vi "Initialise.vi"(8 "error in (no error)":errorcluster, 10 "Message in":refnum<class "InitialiseMessage.lvclass">, 11 "ImageStack in":refnum<class "ImageStack.lvclass">) -> (0 "error out":errorcluster, 3 "ImageStack out":refnum<class "ImageStack.lvclass">)   [LabVIEW 2012, in "ImageStack.lvclass"]
doc: "This method is called when an initialise message is received. It mainly initialises the RabbitMQ connectivity. \n\nOverride this method when your component needs special initialisation (e.g. of software or hardware resources). In that case, don't forget to call the parent for proper implementation. If your component owns subcomponents, they count as resources, so you have to initialise them by calling their own initialise functions"
uses:
  ImageStack.lvclass
  <vilib>/Distrio/Murmex/InitialiseMessage/InitialiseMessage.lvclass
  <vilib>/Distrio/Murmex/Murmex/Murmex.lvclass
  <vilib>/Distrio/Murmex/Murmex/update_cluster.ctl
  <vilib>/Distrio/Murmex/GenericMessage/GenericMessage.lvclass
  <vilib>/Distrio/Murmex/Message/Add or replace parameter.vi
panel:
  # "This method is called when the INTIALISE\ntrigger is sent. \n\nOverride this method when your component needs to\nrespond to this trigger. \n\nCall parent for proper implementation"
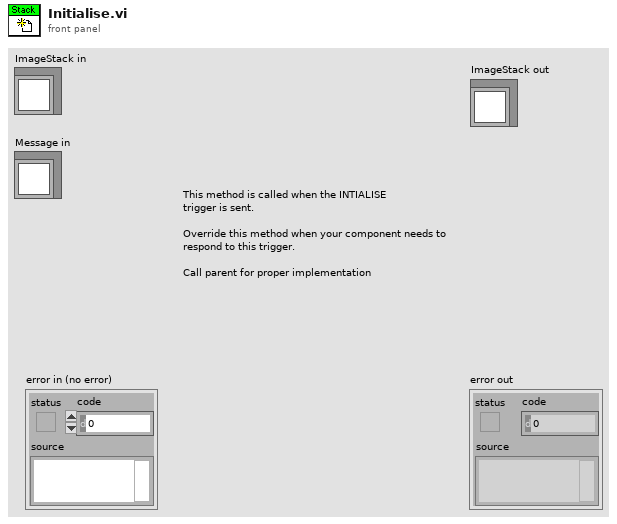
[diagram p1: front panel]
types:
  T1 = typedef "Murmex.lvlib/Murmex.lvclass/update_cluster.ctl" = cluster{"target ID":string, "key chains":string[], "values":variant[]}
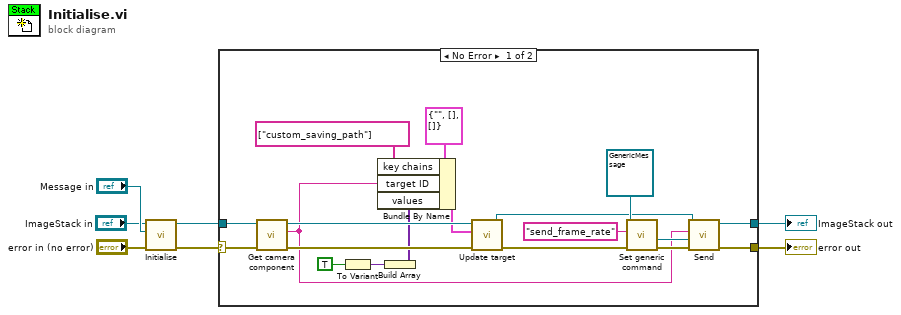
[diagram p0: block diagram]
diagram:
  n1 = call-parent "Initialise.vi"("error in (no error)"="error in (no error)", "Message in"="Message in", "Murmex in"="ImageStack in") -> ("error out"=w4:errorcluster, "Murmex out"=w1:refnum<class "ImageStack.lvclass">)  [unwired: 7 in]
  n2 = case shown="No Error" w4 {
    selector: w4 -> [w26 w28]
    tunnel: [w12 w28] -> w3
    tunnel: [w8 w27] -> w2
    tunnel: w1 -> [w25 w27]
    frame No Error {
      n3 = call-dynamic "Get camera component.vi"("error in (no error)"=w26, "ImageStack in"=w25) -> ("error out"=w24:errorcluster, "Camera component name"=w10:string, "ImageStack out"=w23:refnum<class "ImageStack.lvclass">)  [unwired: 7 in]
      n4 = To Variant(anything=TRUE) -> (Variant=w18:variant)
      n5 = Build Array(w18) -> (w17:variant[])
      n6 = Bundle By Name(cluster=T1 {"target ID"="", "key chains"=[], "values"=[]} ("update cluster"), "key chains"=string[] ["custom_saving_path"], "target ID"=w10, "values"=w17) -> (w21:T1)
      n7 = call <vilib>:"Update target.vi"("error in (no error)"=w24, "update cluster"=w21, "MurmexBase in"=w23) -> ("error out"=w14:errorcluster, "MurmexBase out"=w9:refnum<class "ImageStack.lvclass">)  [unwired: 7 in]
      n8 = call <vilib>:"Set generic command.vi"("error in (no error)"=w14, "generic command"="send_frame_rate", "GenericMessage in"=refnum<class "GenericMessage.lvclass"> refnum ("Distrio Murmex 1.1:GenericMessage")) -> ("error out"=w13:errorcluster, "GenericMessage out"=w11:refnum<class "GenericMessage.lvclass">)  [unwired: 7 in]
      n9 = call <vilib>:"Send.vi"("error in (no error)"=w13, "Message"=w11, "recipient"=w10, "Murmex in"=w9) -> ("error out"=w12:errorcluster, "Murmex out"=w8:refnum<class "ImageStack.lvclass">)  [unwired: 6 in]
    }
    frame Error {
    }
  }
  "error out" <- w3
  "ImageStack out" <- w2
